vi "Dequeue.vi"(8 "error in (no error)":errorcluster, 11 "Masterv2 in":refnum<class "Masterv2.lvclass">) -> (0 "error out":errorcluster, 3 "Masterv2 out":refnum<class "Masterv2.lvclass">, 6 "state":string)   [LabVIEW 2014, in "Main Libraryv2.lvlib" / "Masterv2.lvclass"]
uses:
  Master/Masterv2.lvclass
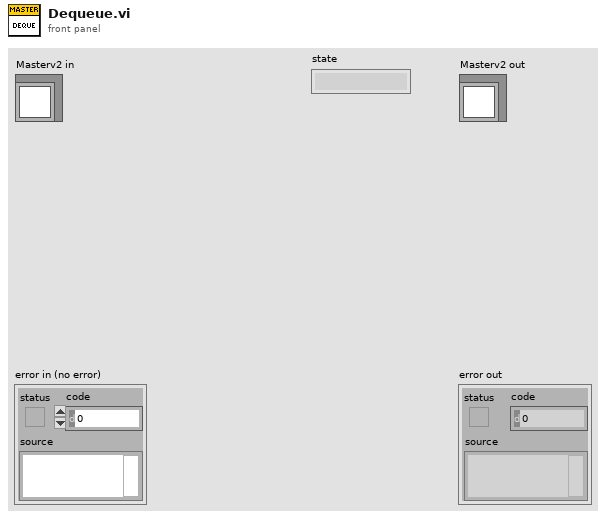
[diagram p1: front panel]
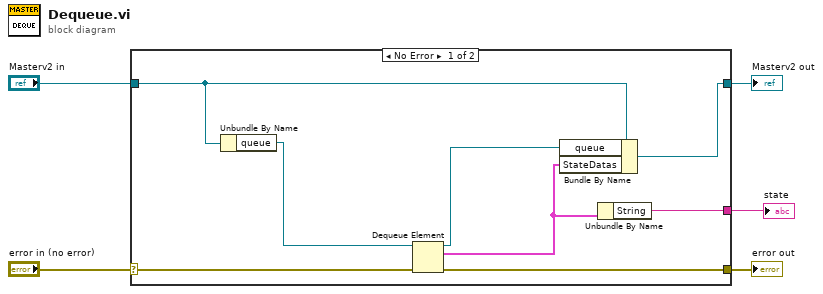
[diagram p0: block diagram]
diagram:
  n1 = case shown="No Error" "error in (no error)" {
    selector: "error in (no error)" -> [w7 w15]
    tunnel: [w6 w15] -> w4
    tunnel: [w13 w14] -> w2
    tunnel: "Masterv2 in" -> [w9 w14]
    tunnel: [w10 _] -> w1
    frame No Error {
      n2 = Unbundle By Name(w9) -> ("queue"=w8:refnum<queue>)
      n3 = Dequeue Element(queue=w8, error in (no error)=w7) -> (queue out=w12:refnum<queue>, element=w11:cluster{"String":string, "Data":variant}, error out=w6:errorcluster)  [unwired: 1 in, 1 out]
      n4 = Bundle By Name(cluster=w9, "queue"=w12, "StateDatas"=w11) -> (w13:refnum<class "Masterv2.lvclass">)
      n5 = Unbundle By Name(w11) -> ("String"=w10:string)
    }
    frame Error {
    }
  }
  "error out" <- w4
  "Masterv2 out" <- w2
  "state" <- w1
